vi "Set AP Sx Sig Curve Val.vi"(6 "yScale":dbl, 7 "numPoints":i32, 8 "error in (no error)":errorcluster caption="错误输入（无错误）", 9 "yArray":dbl, 10 "xArray":dbl, 11 "asicHandle":i32) -> (0 "error out":errorcluster caption="错误输出", 1 "yArray out":dbl, 2 "xArray out":dbl, 3 "function return":i32)   [LabVIEW 2018]
doc: "extern int __stdcall SetAPSxSigCurveVal (int asicHandle, IN double * xArray, IN double * yArray, IN int numPoints, IN double yScale);"
uses:
  APSx.dll/APSx.dll
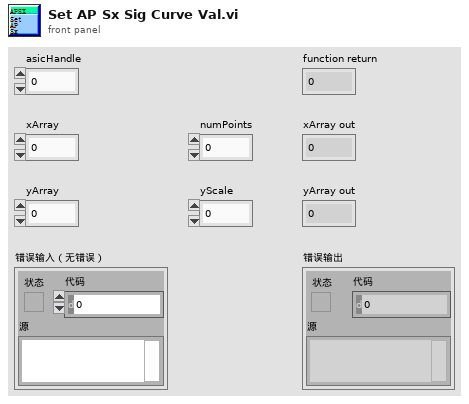
[diagram p1: front panel]
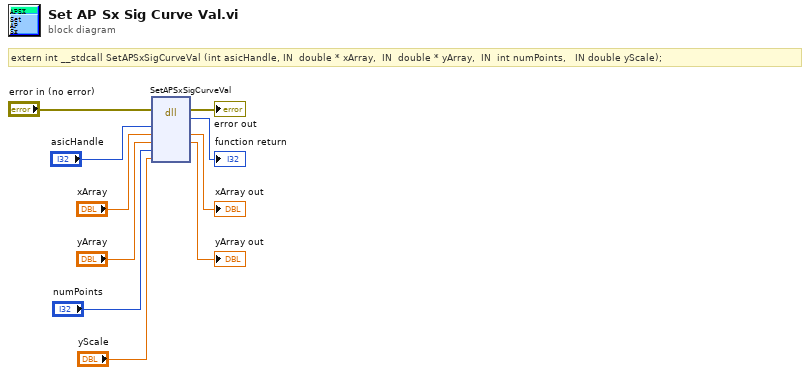
[diagram p0: block diagram]
diagram:
  # "extern int __stdcall SetAPSxSigCurveVal (int asicHandle, IN  double * xArray,  IN  double * yArray,  IN  int numPoints,   IN double yScale);"
  n1 = dll-call lib="PTH2[abs D项目Feng恒隆项目Labview传感器对中台SourcesAPSx.dllAPSx.*" fn="SetAPSxSigCurveVal"(error in="error in (no error)", "asicHandle"="asicHandle", "xArray"="xArray", "yArray"="yArray", "numPoints"="numPoints", "yScale"="yScale") -> (error out=→"error out":errorcluster, →"function return":i32, "xArray"=→"xArray out":dbl, "yArray"=→"yArray out":dbl)  [unwired: 5 in, 1 out]
